vi "Read Frequency Counter.vi"(0 "VISA resource name":refnum<visa-resource-name>, 5 "Marker (0:Marker 1)":i32(ring) items=["Marker 1", "Marker 2", "Marker 3", "Marker 4", "Marker 5", "Marker 6", "Marker 7", "Marker 8", "Marker 9", "Marker 10", "None"], 11 "error in (no error)":errorcluster) -> (4 "VISA resource name out":refnum<visa-resource-name>, 6 "Frequency Counter Output":dbl format="%#_12g", 15 "error out":errorcluster)   [LabVIEW 2020, in "Anritsu Signal Analyzer Series.lvlib"]
doc: "Reads Frequency Counter Data"
uses:
  Anritsu Signal Analyzer Series.lvlib
panel:
  # "Hz"
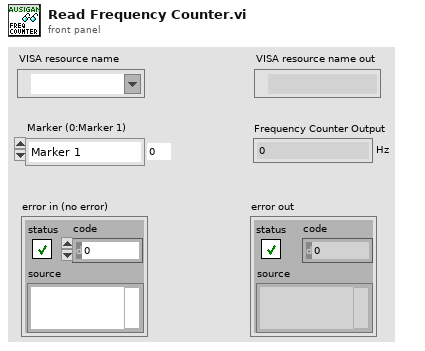
[diagram p1: front panel]
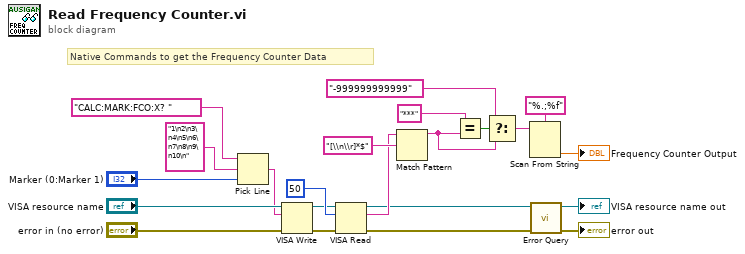
[diagram p0: block diagram]
diagram:
  # "Native Commands to get the Frequency Counter Data"
  n1 = Pick Line(string ("")="CALC:MARK:FCO:X? ", multi-line string="1\n2\n3\n4\n5\n6\n7\n8\n9\n10\n" ("文字列"), line index="Marker (0:Marker 1)") -> (output string=w2:string)
  n2 = VISA Write(VISA resource name="VISA resource name", write buffer=w2, error in (no error)="error in (no error)") -> (VISA resource name out=w7:refnum<visa-resource-name>, error out=w8:errorcluster)  [unwired: 1 out]
  n3 = VISA Read(VISA resource name=w7, byte count=u32 50 ("byte count (0)"), error in (no error)=w8) -> (VISA resource name out=w6:refnum<visa-resource-name>, read buffer=w15:string, error out=w5:errorcluster)  [unwired: 1 out]
  n4 = Match Pattern(string=w15, regular expression="[\\n\\r]*$") -> (before substring=w17:string)  [unwired: 1 in, 3 out]
  n5 = Equal?(x="***", y=w17) -> (x = y?=w12:bool)
  n6 = Select(t="-999999999999", s=w12, f=w17) -> (s? t:f=w13:string)
  n7 = Scan From String(format string="%.;%f" ("形式文字列"), input string=w13) -> (output 1=→"Frequency Counter Output":dbl)  [unwired: 3 in, 3 out]
  n8 = call "Error Query.vi"("error in (no error)"=w5, "VISA resource name"=w6) -> ("error out"=→"error out":errorcluster, "VISA resource name out"=→"VISA resource name out":refnum<visa-resource-name>)  [unwired: 6 in, 2 out]
